vi "poly_timing_tools_eco_minus.vi"(4 "code (w/ eco)":i32) -> (1 "code (- eco)":i32)   [LabVIEW 2015, in "_timing_tools_polys.lvlib"]
uses:
  _timing_tools_polys.lvlib
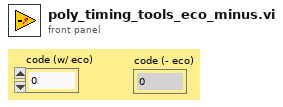
[diagram p1: front panel]
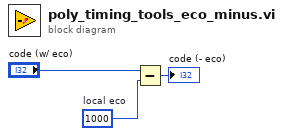
[diagram p0: block diagram]
diagram:
  w1 = 1000  # local eco
  n1 = Subtract(x="code (w/ eco)", y=w1) -> (x-y=→"code (- eco)":i32)
